vi "Global 1.vi"() -> ()   [LabVIEW 2016]
panel:
  in  "offset X":dbl
  in  "offset Y":dbl
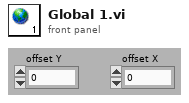
[diagram p1: front panel]
diagram:
